vi "Write Server Controller Enqueuer.vi"(8 "error in (no error)":errorcluster, 10 "Actor Framework:Message Enqueuer":refnum<class "Message Enqueuer.lvclass">, 11 "WS Server in":refnum<class "WS Server.lvclass">) -> (0 "error out":errorcluster, 3 "WS Server out":refnum<class "WS Server.lvclass">)   [LabVIEW 2016, in "WebSocket Networking.lvlib" / "WS Server.lvclass"]
uses:
  <userlib>/Common Components/WebSocket Networking/WS Server/WS Server.lvclass
  <vilib>/ActorFramework/Message Enqueuer/Message Enqueuer.lvclass
  <userlib>/Common Components/WebSocket Networking/WS Server/WS Server.lvclass/WS Server.ctl
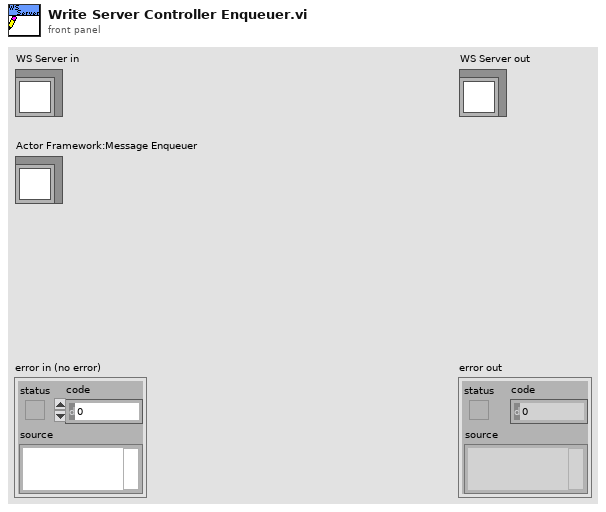
[diagram p1: front panel]
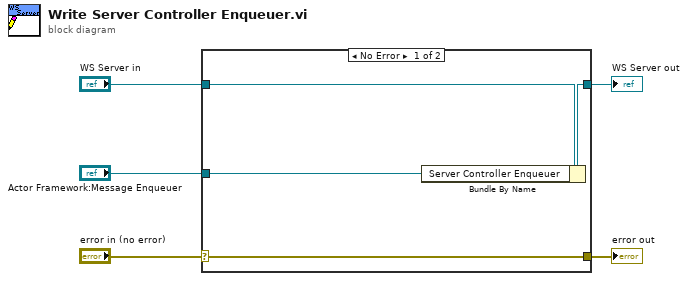
[diagram p0: block diagram]
diagram:
  n1 = case shown="No Error" "error in (no error)" {
    selector: "error in (no error)" -> [w9 w10]
    tunnel: [w9 w10] -> w4
    tunnel: [w7 w11] -> w2
    tunnel: "WS Server in" -> [w8 w11]
    tunnel: "Actor Framework:Message Enqueuer" -> [w6 _]
    frame No Error {
      n2 = Bundle By Name(cluster=w8, "Server Controller Enqueuer"=w6) -> (w7:refnum<class "WS Server.lvclass">)
    }
    frame Error {
    }
  }
  "error out" <- w4
  "WS Server out" <- w2
